vi "LVFPGA full duplex.vi"(0 "device name":string="RIO0", 1 "Enabled Channels":string(combo)="0", 5 "IQ rate":dbl=10000000.0 caption="IQ Rate" format="%#.3pS/s", 7 "number of samples":i64=16384 caption="Number of Samples", 9 "run duration":dbl=5.0 format="%#_13g", 11 "error in":errorcluster) -> (6 "Coerced IQ Rate":dbl format="%#_6p", 8 "underflow":bool, 10 "overflow":bool, 15 "error out":errorcluster)   [LabVIEW 2014]
doc: "This template is for the Simple NI-USRP Streaming design, a design that shows the basics of streaming data to and from an NI USRP-294x/295x device. Refer to the block diagram for more information about how to use this template."
uses:
  subVIs/Start Trigger.ctl
  subVIs/Configure Signal (Level).vi
  subVIs/Write Tx Data (I16 multi).vi
  subVIs/Fetch Rx Data (1D CDB WDT).vi
panel:
  out "generating":bool caption="Generating"
  in  "stop":bool
  # "Full Duplex Streaming"
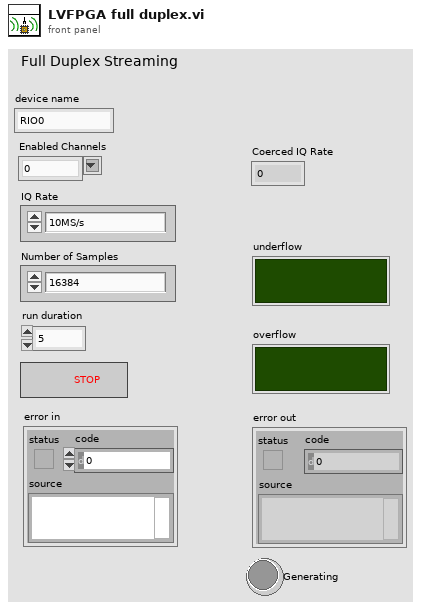
[diagram p1: front panel]
types:
  T1 = typedef "niUsrpRio Config v1 Host.lvlib/niUsrpRio Session.ctl" = cluster{"Global Settings Register Bus":T2, "Radio 0 Settings Register Bus":T2, "FPGA Interface":refnum<k20>, "RIO Interface Number":u32, "EEPROM Header":T3, "Device Data Header":T4, "EEPROM Characterization Header":T5, "Characterization Data":T6[], "Characterization Data Valid?":bool, "Radio 1 Settings Register Bus":T2, "Radio Settings Bus Semaphore":T8, "FPGA Current Version":u32, "FPGA Oldest Compatible Version":u32, "Fixed Logic Current Version":u32, "Fixed Logic Oldest Compatible Version":u32, "FPGA Radio Settings Bus Current Version":u32, "FPGA Radio Settings Bus Oldest Compatible Version":u32, "DB 0":T9, "DB 1":T9}
  T2 = typedef "niInstr Register Bus v0 Host.lvlib/Register Bus Session.ctl" = refnum<queue>
  T3 = typedef "niUsrpRio Config v1 Host.lvlib/EEPROM Header.ctl" = cluster{"Checksum":u32, "Product Code":u16, "Hardware Current Version":u16, "Hardware Oldest Compatible Version":u16, "EEPROM Map Current Version":u16, "EEPROM Map Oldest Compatible Version":u16, "User Password":string, "Pointer to Factory Header":u32, "Pointer to User Header":u32, "Recommended Interval":u16, "Number of Reserved Bytes":i32, "Number of Daughterboards":u8, "Daughterboard IDs":u16[], "Daughterboard Serial Numbers":string[]}
  T4 = typedef "niUsrpRio Config v1 Host.lvlib/EEPROM Device Data Header.ctl" = cluster{"Checksum":u32, "Number of Channels":u8, "Number of Gain Settings":u16[], "Pointer to Characterization Data":u32[], "Number of Reserved Bytes":i32, "Number of Frequencies":u16[]}
  T5 = typedef "niUsrpRio Config v1 Host.lvlib/EEPROM Characterization Header.ctl" = cluster{"Checksum":u32, "Date":timestamp, "Temperature":sgl, "Misc. Info":string, "Pointer to Device Data Header":u32, "Number of Reserved Bytes":i32}
  T6 = typedef "niUsrpRio Config v1 Host.lvlib/Characterization Data.ctl" = cluster{"Gains[dB]":dbl[], "Frequencies [Hz]":dbl[], "IQ Imbalance Table":T7[], "Measured Gains[dB]":dbl[][]}
  T7 = typedef "niUsrpRio Config v1 Host.lvlib/IQ Imbalance.ctl" = cluster{"Gain Imbalance [linear]":dbl, "Phase Imbalance [radians]":dbl, "Offset":cdb}
  T8 = typedef "Semaphore RefNum" = refnum<k1>
  T9 = typedef "niUsrpRio Config v1 Host.lvlib/DB settings.ctl" = cluster{"Register Settings Bus Duplex SBX CBX":T10, "Register Settings Bus  Idle SBX CBX":T10, "Register Settings Bus Rx SBX CBX":T10, "Register Settings Bus Tx SBX CBX":T10, "Register Settings Bus Duplex WBX":T11, "Register Settings Bus Idle WBX":T11, "Register Settings Bus Rx WBX":T11, "Register Settings Bus Tx WBX":T11, "ADF4351 Registers Rx":T12, "ADF4351 Registers Tx":T12, "MAX2870 Register Rx":T19, "MAX2870 Register Tx":T19}
  T10 = typedef "niUsrpRio Config v1 Host.lvlib/ATR Register Settings SBX CBX.ctl" = cluster{"TX LO LPF":bool, "TX/RX Switch":bool, "TX ATTN":dbl, "TX Ant Selection":bool, "TX Lock Detect":bool, "Disable TX Power":bool, "TX Enabled":bool, "PLL CE TX":bool, "PLL PDBrf TX":bool, "PLL MUXOUT TX":bool, "PLL Lock Detect TX":bool, "RX LO LPF":bool, "LNA Switch":bool, "RX ATTN":dbl, "RX Ant Selection":bool, "RX Lock Detect":bool, "Disable RX Power":bool, "RX Disable":bool, "PLL CE RX":bool, "PLL PDBrf RX":bool, "PLL MUXOUT RX":bool, "PLL Lock Detect RX":bool, "Cached Value":u32, "Cached Rx Gain":dbl}
  T11 = typedef "niUsrpRio Config v1 Host.lvlib/ATR Register Settings WBX.ctl" = cluster{"TX/RX Ant Select":bool, "TX 5V Supply":bool, "TX 3.3V Supply":bool, "TX ATTN":dbl, "TX PLL PDBrf":bool, "TX PLL Lock Detect":bool, "RX1/RX2":bool, "RX ATTN":dbl, "RX 5V Supply":bool, "RX 3.3V Supply":bool, "Baseband":bool, "RX PLL CE":bool, "RX PLL PDBrf":bool, "RX PLL MUXOUT":bool, "RX PLL Lock Detect":bool, "Cached Value":u32, "Cached RX Gain":dbl}
  T12 = typedef "niUsrpRio Config v1 Host.lvlib/ADF4351_Registers.ctl" = cluster{"Register 0":T13, "Register 1":T14, "Register 2":T15, "Register 3":T16, "Register 4":T17, "Register 5":T18, "update":bool}
  T13 = typedef "niUsrpRio Config v1 Host.lvlib/ADF4351_Register0.ctl" = cluster{"INT":u16, "FRAC":u16, "C3":bool, "C2":bool, "C1":bool}
  T14 = typedef "niUsrpRio Config v1 Host.lvlib/ADF4351_Register1.ctl" = cluster{"PHASE ADJUST":bool, "PRESCALAR":bool, "PHASE":u16, "MOD":u16, "C3":bool, "C2":bool, "C1":bool}
  T15 = typedef "niUsrpRio Config v1 Host.lvlib/ADF4351_Register2.ctl" = cluster{"LOW NOISE AND LOW SPUR ":u8, "MUXOUT":u8, "REF DBLR":bool, "RDIV2":bool, "10-bit R COUNTER":u16, "DOUBLE BUFFER":bool, "CHARGE PUMP CURRENT SETTING":u8, "LDF":bool, "LDP":bool, "PD POLARITY":bool, "POWER DOWN":bool, "CP THREE-STATE":bool, "COUNTER RESET":bool, "C3":bool, "C2":bool, "C1":bool}
  T16 = typedef "niUsrpRio Config v1 Host.lvlib/ADF4351_Register3.ctl" = cluster{"BAND SELECT CLOCK MODE":bool, "ABP":bool, "CHARGE CANCEL":bool, "CSR":bool, "CLK DIV MODE":u8, "CLK DIV VAL":u16, "C3":bool, "C2":bool, "C1":bool}
  T17 = typedef "niUsrpRio Config v1 Host.lvlib/ADF4351_Register4.ctl" = cluster{"FEEDBACK \nSELECT":bool, "RF DIVIDER SEL":u8, "BAND SELECT\nCLK DIV VAL":u8, "VCO PWR DWN":bool, "Mute Till Lock Detect":bool, "AUX OUT SEL":bool, "AUX OUT EN":bool, "AUX OUT PWR":u8, "RF OUT EN":bool, "OUTPUT PWR":u8, "C3":bool, "C2":bool, "C1":bool}
  T18 = typedef "niUsrpRio Config v1 Host.lvlib/ADF4351_Register5.ctl" = cluster{"LD PIN MODE":u8, "C3":bool, "C2":bool, "C1":bool}
  T19 = typedef "niUsrpRio Config v1 Host.lvlib/MAX2870_Synthesizer.ctl" = cluster{"Register 0":T20, "Register 1":T21, "Register 2":T22, "Register 3":T23, "Register 4":T24, "Register 5":T25, "update":bool}
  T20 = typedef "niUsrpRio Config v1 Host.lvlib/MAX2870_Register0.ctl" = cluster{"INT mode":bool, "INT":u16, "FRAC":u16, "C3":bool, "C2":bool, "C1":bool}
  T21 = typedef "niUsrpRio Config v1 Host.lvlib/MAX2870_Register1.ctl" = cluster{"CPOC":bool, "CPL":u8, "CPT":u8, "PHASE":u16, "MOD":u16, "C3":bool, "C2":bool, "C1":bool}
  T22 = typedef "niUsrpRio Config v1 Host.lvlib/MAX2870_Register2.ctl" = cluster{"LDS":bool, "SDN":u8, "MUX":u8, "DBR":bool, "RDIV2":bool, "R":u16, "REG4DB":bool, "CP":u8, "LDF":bool, "LDP":bool, "PDP":bool, "SHDN":bool, "TRI":bool, "RST":bool, "C3":bool, "C2":bool, "C1":bool}
  T23 = typedef "niUsrpRio Config v1 Host.lvlib/MAX2870_Register3.ctl" = cluster{"VCO":u8, "VAS_SHDN":bool, "RETUNE":bool, "CDM":u8, "CDIV":u16, "C3":bool, "C2":bool, "C1":bool}
  T24 = typedef "niUsrpRio Config v1 Host.lvlib/MAX2870_Register4.ctl" = cluster{"FB":bool, "DIVA":u8, "BS":u16, "BDIV":bool, "RFB_EN":bool, "BPWR":u8, "RFA_EN":bool, "APWR":u8, "C3":bool, "C2":bool, "C1":bool}
  T25 = typedef "niUsrpRio Config v1 Host.lvlib/MAX2870_Register5.ctl" = cluster{"F01":bool, "LD":u8, "MUX":bool, "C3":bool, "C2":bool, "C1":bool}
  T26 = cluster{"antenna":string, "frequency":dbl, "lo frequency":dbl, "level":dbl}[]
  T27 = typedef "Start Trigger.ctl" = enum8{"Software", "Digital Edge", "Rx Start Trigger", "Tx Start Trigger", "Immediate"}
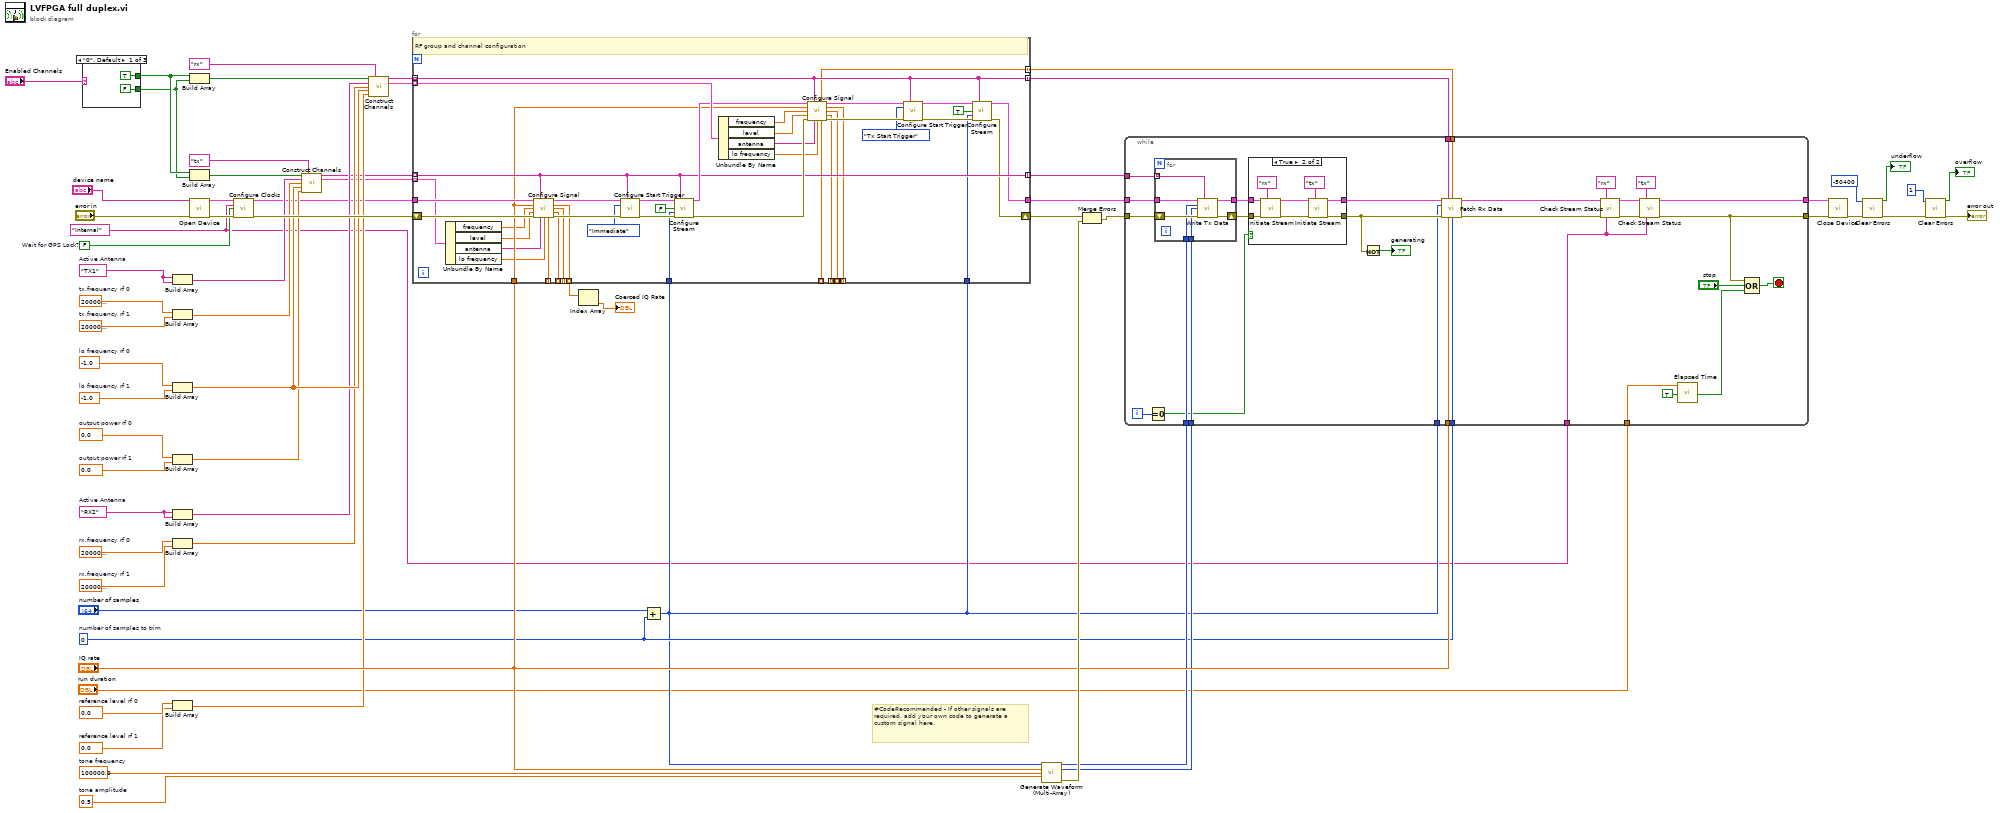
[diagram p0: block diagram]
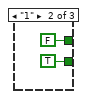
[diagram p2: hidden frame]
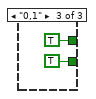
[diagram p3: hidden frame]
diagram:
  w60 = 100000.0  # tone frequency
  w47 = 0.0  # reference level rf 1
  w48 = 0.0  # reference level rf 0
  w51 = 2000000000.0  # rx.frequency rf 1
  w52 = 2000000000.0  # rx.frequency rf 0
  w39 = 0.0  # output power rf 1
  w40 = 0.0  # output power rf 0
  w49 = -1.0  # lo frequency rf 1
  w50 = -1.0  # lo frequency rf 0
  w41 = 2000000000.0  # tx.frequency rf 1
  w42 = 2000000000.0  # tx.frequency rf 0
  w10 = "Internal" ("reference frequency source")
  w18 = u32 0  # number of samples to trim
  w33 = "TX1"  # Active Antenna
  w34 = "RX2"  # Active Antenna
  w59 = 0.5  # tone amplitude
  w57 = FALSE  # Wait for GPS Lock?
  # "#CodeRecommended - If other signals are required, add your own code to generate a custom signal here."
  n1 = case shown="\"0\", Default" "Enabled Channels" {
    tunnel: [TRUE FALSE TRUE] -> w15
    tunnel: [FALSE TRUE TRUE] -> w14
    frame "0", Default {
    }
    frame "1" {
    }
    frame "0,1" {
    }
  }
  n2 = Build Array(w33, w33) -> (w27:string[])
  n3 = Build Array(w42, w41) -> (w31:dbl[])
  n4 = Build Array(w50, w49) -> (w32:dbl[])
  n5 = Build Array(w40, w39) -> (w29:dbl[])
  n6 = Build Array(w34, w34) -> (w26:string[])
  n7 = Build Array(w52, w51) -> (w30:dbl[])
  n8 = Build Array(w48, w47) -> (w28:dbl[])
  n9 = Build Array(w15, w14) -> (w56:bool[])
  n10 = Build Array(w15, w14) -> (w55:bool[])
  n11 = call "Open Device.vi"("USRP RIO device"="device name", "error in"="error in") -> ("niUsrpRio Session (out)"=w43:T1, "error out"=w64:errorcluster)  [unwired: 12 in]
  n12 = call "Configure Clocks.vi"("niUsrpRio Session"=w43, "Reference Frequency Source"=w10, "Wait for GPS Lock?"=w57, "error in"=w64) -> ("niUsrpRio Session (out)"=w25:T1, "error out"=w53:errorcluster)  [unwired: 10 in]
  n13 = call "Construct Channels.vi"("enabled channels"=w55, "scope"="tx", "antennas"=w27, "frequencies"=w31, "lo frequencies"=w32, "levels"=w29) -> ("channels"=w24:string[], "channel configurations"=w22:T26)  [unwired: 8 in]
  n14 = call "Construct Channels.vi"("enabled channels"=w56, "scope"="rx", "antennas"=w26, "frequencies"=w30, "lo frequencies"=w32, "levels"=w28) -> ("channels"=w35:string[], "channel configurations"=w23:T26)  [unwired: 8 in]
  n15 = Add(x="number of samples", y=w18) -> (x+y=w17:i64)
  n16 = for {
    tunnel: [w86] -> _ mode=indexing
    tunnel: w25 -> [w97]
    tunnel: w35 -> [w96] mode=indexing
    tunnel: w24 -> [w110] mode=indexing
    tunnel: [w87] -> w37
    tunnel: "IQ rate" -> [w78]
    tunnel: w17 -> [w99]
    tunnel: w17 -> [w98]
    shift-right: [w109] -> w38
    shift-left: w53 -> [w100]
    tunnel: [w110] -> w36 mode=indexing
    tunnel: [w96] -> w44 mode=indexing
    tunnel: [w95] -> w46 mode=indexing
    tunnel: [w94] -> _ mode=indexing
    tunnel: [w93] -> _ mode=indexing
    tunnel: [w92] -> w2 mode=indexing
    tunnel: [w91] -> _ mode=indexing
    tunnel: [w90] -> _ mode=indexing
    tunnel: [w89] -> _ mode=indexing
    tunnel: [w88] -> _ mode=indexing
    tunnel: w23 -> [w113] mode=indexing
    tunnel: w22 -> [w79] mode=indexing
    # "RF group and channel configuration"
    n17 = Unbundle By Name(w79) -> ("frequency"=w77:dbl, "level"=w76:dbl, "antenna"=w75:string, "lo frequency"=w74:dbl)
    n18 = call-poly "Configure Signal.vi"("niUsrpRio Session"=w97, "scope"=w110, "sample rate [S/s]"=w78, "frequency [Hz]"=w77, "level [dBm]"=w76, "error in"=w100, "Active Antenna"=w75, "LO frequency [Hz]"=w74) -> ("niUsrpRio Session (out)"=w106:T1, "coerced sample rate [S/s]"=w92:dbl, "coerced frequency [Hz]"=w93:dbl, "coerced level [dBm]"=w94:dbl, "coerced LO frequency [Hz]"=w86:dbl, "error out"=w108:errorcluster)  [unwired: 1 in, 1 out]
    n19 = call "Configure Start Trigger.vi"("niUsrpRio Session"=w106, "scope"=w110, "start trigger"=Start_Trigger."Immediate" ("tx.start trigger"), "error in"=w108) -> ("niUsrpRio Session (out)"=w105:T1, "error out"=w107:errorcluster)  [unwired: 10 in]
    n20 = call "Configure Stream.vi"("niUsrpRio Session"=w105, "scope"=w110, "number of samples is finite"=FALSE, "number of samples"=w99, "error in"=w107) -> ("niUsrpRio Session (out)"=w112:T1, "error out"=w111:errorcluster)  [unwired: 9 in]
    n21 = Unbundle By Name(w113) -> ("frequency"=w83:dbl, "level"=w82:dbl, "antenna"=w81:string, "lo frequency"=w80:dbl)
    n22 = call-poly "Configure Signal.vi"("niUsrpRio Session"=w112, "scope"=w96, "sample rate [S/s]"=w78, "frequency [Hz]"=w83, "level [dBm]"=w82, "error in"=w111, "Active Antenna"=w81, "LO frequency [Hz]"=w80) -> ("coerced vertical range [Vpp]"=w95:dbl, "niUsrpRio Session (out)"=w102:T1, "coerced sample rate [S/s]"=w88:dbl, "coerced frequency [Hz]"=w89:dbl, "coerced level [dBm]"=w90:dbl, "coerced LO frequency [Hz]"=w91:dbl, "error out"=w103:errorcluster)  [unwired: 1 in]
    n23 = call "Configure Start Trigger.vi"("niUsrpRio Session"=w102, "scope"=w96, "start trigger"=Start_Trigger."Tx Start Trigger" ("rx.start trigger"), "error in"=w103) -> ("niUsrpRio Session (out)"=w101:T1, "error out"=w104:errorcluster)  [unwired: 10 in]
    n24 = call "Configure Stream.vi"("niUsrpRio Session"=w101, "scope"=w96, "number of samples is finite"=TRUE, "number of samples"=w98, "error in"=w104) -> ("niUsrpRio Session (out)"=w87:T1, "error out"=w109:errorcluster)  [unwired: 9 in]
  }
  n25 = Index Array(array=w2) -> (element=→"Coerced IQ Rate":dbl)  [unwired: 1 in]
  n26 = call "Generate Waveform (Multi-Array).vi"("number of samples"=w17, "sample rate"="IQ rate", "tone frequency"=w60, "amplitude"=w59) -> ("I"=w20:i16[], "Q"=w19:i16[], "error out"=w65:errorcluster)  [unwired: 8 in, 1 out]
  n27 = Merge Errors(w38, w65) -> (w63:errorcluster)
  n28 = while {
    tunnel: w37 -> [w126]
    tunnel: [w131] -> w62
    tunnel: w46 -> [w142]
    tunnel: "IQ rate" -> [w141]
    tunnel: w17 -> [w140]
    tunnel: w44 -> [w139]
    tunnel: w63 -> [w127]
    tunnel: [w134] -> w61
    tunnel: w18 -> [w128]
    tunnel: w20 -> [w123]
    tunnel: w19 -> [w122]
    tunnel: w36 -> [w121]
    tunnel: "run duration" -> [w117]
    tunnel: w10 -> [w116]
    i -> [w115]
    stop <- w129 stop-if-true
    # "Acquire and Fetch a waveform"
    n29 = Equal To 0?(x=w115) -> (x = 0?=w114:bool)
    n30 = for {
      tunnel: w126 -> [w159]
      shift-right: [w160] -> w125
      shift-left: w127 -> [w161]
      tunnel: [w158] -> w124
      tunnel: w122 -> [w157]
      tunnel: w123 -> [w156]
      tunnel: w121 -> [w155] mode=indexing
      n31 = call-poly "Write Tx Data.vi"("niUsrpRio Session"=w159, "scope"=w155, "I"=w156, "Q"=w157, "error in"=w161) -> ("niUsrpRio Session (out)"=w158:T1, "error out"=w160:errorcluster)  [unwired: 9 in]
    }
    n32 = case shown="True" w114 {
      tunnel: [w145 w154] -> w144
      tunnel: [w146 w153] -> w135
      tunnel: w125 -> [w145 w152]
      tunnel: w124 -> [w146 w151]
      frame False {
      }
      frame True {
        n33 = call "Initiate Stream.vi"("niUsrpRio Session"=w151, "scope"="rx", "error in"=w152) -> ("niUsrpRio Session (out)"=w149:T1, "error out"=w150:errorcluster)  [unwired: 11 in]
        n34 = call "Initiate Stream.vi"("niUsrpRio Session"=w149, "scope"="tx", "error in"=w150) -> ("niUsrpRio Session (out)"=w153:T1, "error out"=w154:errorcluster)  [unwired: 11 in]
      }
    }
    n35 = Not(x=w144) -> (.not. x?=→"generating":bool)
    n36 = call-poly "Fetch Rx Data.vi"("niUsrpRio Session"=w135, "scope"=w139, "vertical ranges [Vpp]"=w142, "number of samples"=w140, "error in"=w144, "sample rate"=w141, "leading samples to trim"=w128) -> ("niUsrpRio Session (out)"=w138:T1, "error out"=w143:errorcluster)  [unwired: 6 in, 1 out]
    n37 = call "Check Stream Status.vi"("niUsrpRio Session"=w138, "scope"="rx", "error in"=w143, "reference frequency source"=w116) -> ("niUsrpRio Session (out)"=w132:T1, "error out"=w133:errorcluster)  [unwired: 9 in, 1 out]
    n38 = call "Check Stream Status.vi"("niUsrpRio Session"=w132, "scope"="tx", "error in"=w133, "reference frequency source"=w116) -> ("niUsrpRio Session (out)"=w131:T1, "error out"=w134:errorcluster)  [unwired: 9 in, 1 out]
    n39 = call "Elapsed Time"("Time Target (s)"=w117, "Auto Reset"=TRUE) -> ("Time has Elapsed"=w118:bool)  [unwired: 10 in, 7 out]
    n40 = Compound Arithmetic op=OR(w134, "stop", w118) -> (w129:bool)
  }
  n41 = call "Close Device.vi"("niUsrpRio Session"=w62, "error in"=w61) -> ("error out"=w9:errorcluster)  [unwired: 13 in]
  n42 = call <vilib>:"Clear Errors.vi"("error in (no error)"=w9, "specific error code to clear (0: all)"=-50400) -> ("error out"=w6:errorcluster, "specific error cleared?"=→"underflow":bool)  [unwired: 4 in]
  n43 = call <vilib>:"Clear Errors.vi"("error in (no error)"=w6, "specific error code to clear (0: all)"=1) -> ("error out"=→"error out":errorcluster, "specific error cleared?"=→"overflow":bool)  [unwired: 4 in]
